vi "DSF.Execution.Runtime.Plugin Manager.Objects to Plugin.vi"(8 "error in (no error)":errorcluster, 10 "Plugin objects":refnum<class>[](array[class]), 11 "Plugin Manager in":refnum<class "DSF.Engine.Runtime.Plugin Manager.lvclass">) -> (0 "error out":errorcluster, 2 "Plugin":refnum<class "DSF.Engine.Plugin.lvclass">, 3 "Plugin Manager out":refnum<class "DSF.Engine.Runtime.Plugin Manager.lvclass">)   [LabVIEW 2017, in "DSF.Engine.lvlib" / "DSF.Engine.Runtime.Plugin Manager.lvclass"]
uses:
  DSF.Engine.Runtime.Plugin Manager.lvclass
  Shared/Classes/Plugin/DSF.Shared.Configuration.Plugin.lvclass
  Shared/Classes/Transfer Group/DSF.Shared.Configuration.Transfer Group.lvclass
  Shared/Classes/Transfer/DSF.Shared.Configuration.Transfer.lvclass
  Shared/Typedefs/DSF.Shared.Typedefs.Plugin Classes.Configuration.ctl
  DSF.Shared.lvlib
  Plugin/DSF.Engine.Plugin.Runtime.lvclass
  Shared/Typedefs/DSF.Shared.Typedefs.Plugin Classes.Runtime.ctl
  Shared/Typedefs/DSF.Shared.Typedefs.Plugin Classes.ctl
  Plugin/DSF.Engine.Plugin.lvclass
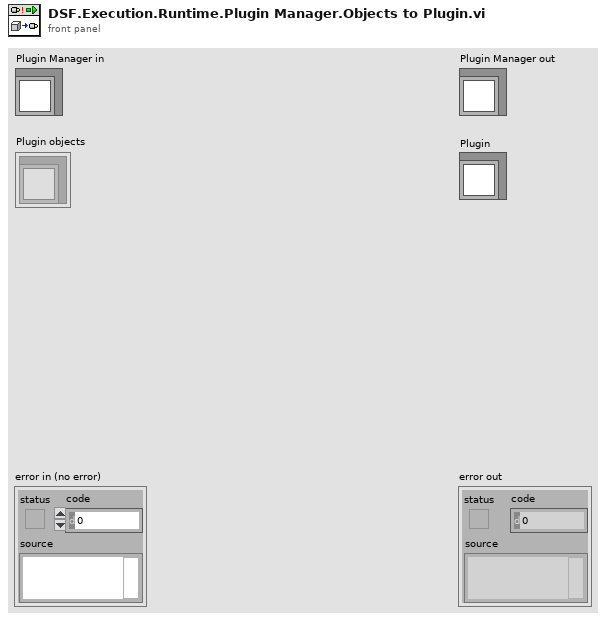
[diagram p1: front panel]
types:
  T1 = typedef "DSF.Shared.lvlib/DSF.Shared.Typedefs.Plugin Classes.ctl" = cluster{"Configuration":T2, "Runtime":T3}
  T2 = typedef "DSF.Shared.lvlib/DSF.Shared.Typedefs.Plugin Classes.Configuration.ctl" = cluster{"Plugin":refnum<class "DSF.Shared.Configuration.Plugin.lvclass">, "Transfer Group":refnum<class "DSF.Shared.Configuration.Transfer Group.lvclass">, "Transfer":refnum<class "DSF.Shared.Configuration.Transfer.lvclass">}
  T3 = typedef "DSF.Shared.lvlib/DSF.Shared.Typedefs.Plugin Classes.Runtime.ctl" = cluster{"Plugin":refnum<class "DSF.Engine.Plugin.Runtime.lvclass">}
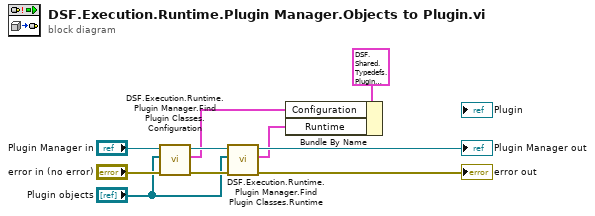
[diagram p0: block diagram]
diagram:
  n1 = call "DSF.Execution.Runtime.Plugin Manager.Find Plugin Classes.Configuration.vi"("error in (no error)"="error in (no error)", "Plugin objects"="Plugin objects", "Plugin Manager in"="Plugin Manager in") -> ("error out"=w7:errorcluster, "Plugin Configuration Classes"=w5:T2, "Plugin Manager out"=w8:refnum<class "DSF.Engine.Runtime.Plugin Manager.lvclass">)  [unwired: 6 in]
  n2 = call "DSF.Execution.Runtime.Plugin Manager.Find Plugin Classes.Runtime.vi"("error in (no error)"=w7, "Plugin objects"="Plugin objects", "Plugin Manager in"=w8) -> ("error out"=→"error out":errorcluster, "Plugin Runtime Classes"=w2:T3, "Plugin Manager out"=→"Plugin Manager out":refnum<class "DSF.Engine.Runtime.Plugin Manager.lvclass">)  [unwired: 6 in]
  n3 = Bundle By Name(cluster=T1 {"Configuration"={"Plugin"=refnum, "Transfer Group"=refnum, "Transfer"=refnum}, "Runtime"={"Plugin"=refnum}} ("Plugin Classes"), "Configuration"=w5, "Runtime"=w2) -> ()  [unwired: 1 out]
